vi "Square Pulse Fit Result String.vi"(8 "error in (no error)":errorcluster, 9 "Square Pulse Statistics":T3 {"Falling Edge Width" format="%0.2f"; "Rising Edge Width" format="%0.2f"; "Falling Edge Midpoint" format="%0.2f"; "Rising Edge Midpoint" format="%0.2f"; "Low Level" format="%0.2f"; "High Level" format="%0.2f"}, 10 "Square Pulse Options":T1={"Method"=enum."Mode", "# Bins"=0, "Threshold %"=10.0, "Center on Midpoint"=FALSE, "Smoothen Plot"=FALSE}, 11 "ROI Descriptor":T4 {"Contours"."Type" items=["No Selection", "Point", "Line", "Rectangle", "Oval", "Polygon", "Freehand Region", "Annulus", "Unused2", "Unused3", "Broken Line", "Freehand Line", "Rotated Rectangle"]}) -> (0 "error out":errorcluster, 3 "Result String":string)   [LabVIEW 2021, in "Fits.lvlib"]
uses:
  Fits.lvlib
  Square Pulse Statistics.ctl
  Square Pulse Options.ctl
  Square Pulse Levels Type.ctl
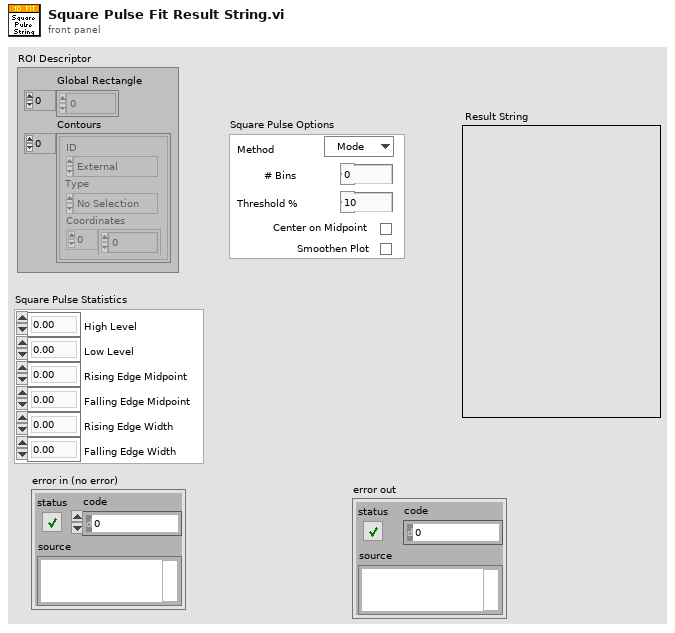
[diagram p1: front panel]
types:
  T1 = typedef "Fits.lvlib/Square Pulse Options.ctl" = cluster{"Method":T2, "# Bins":i32, "Threshold %":dbl, "Center on Midpoint":bool, "Smoothen Plot":bool}
  T2 = typedef "Fits.lvlib/Square Pulse Levels Type.ctl" = enum16{"Mode", "Mean"}
  T3 = typedef "Fits.lvlib/Square Pulse Statistics.ctl" = cluster{"High Level":dbl, "Low Level":dbl, "Rising Edge Midpoint":dbl, "Falling Edge Midpoint":dbl, "Rising Edge Width":dbl, "Falling Edge Width":dbl}
  T4 = typedef "ROI Descriptor" = cluster{"Global Rectangle":i32[], "Contours":cluster{"ID":enum32{"External", "Internal"}, "Type":u32, "Coordinates":i32[]}[]}
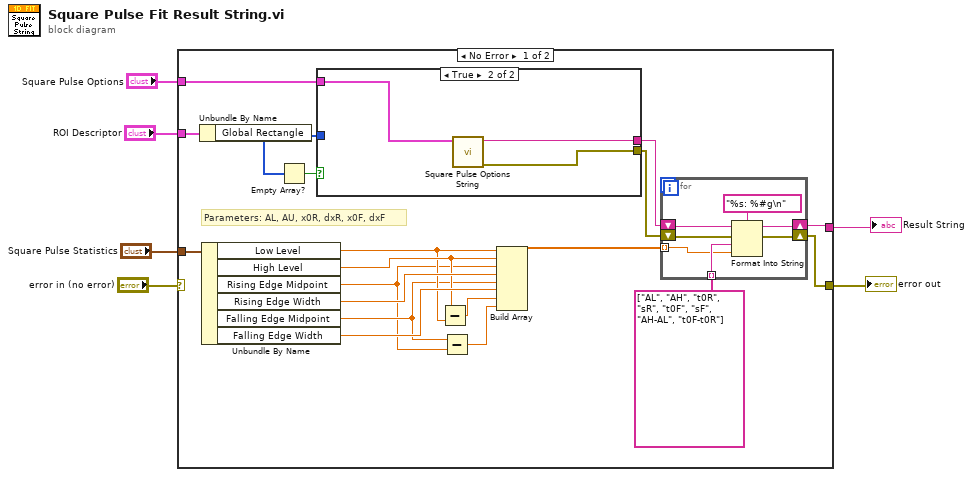
[diagram p0: block diagram]
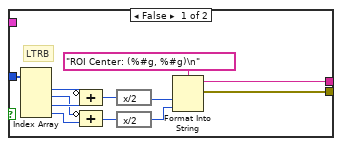
[diagram p2: hidden frame]
diagram:
  n1 = case shown="No Error" "error in (no error)" {
    selector: "error in (no error)" -> [_ w48]
    tunnel: [w21 w48] -> w5
    tunnel: "ROI Descriptor" -> [w25 _]
    tunnel: [w22 _] -> w3
    tunnel: "Square Pulse Statistics" -> [w17 _]
    tunnel: "Square Pulse Options" -> [w7 _]
    frame No Error {
      # "Parameters: AL, AU, x0R, dxR, x0F, dxF"
      n2 = Unbundle By Name(w25) -> ("Global Rectangle"=w20:i32[])
      n3 = Unbundle By Name(w17) -> ("Low Level"=w12:dbl, "High Level"=w13:dbl, "Rising Edge Midpoint"=w9:dbl, "Rising Edge Width"=w16:dbl, "Falling Edge Midpoint"=w10:dbl, "Falling Edge Width"=w15:dbl)
      n4 = Empty Array?(array=w20) -> (empty?=w19:bool)
      n5 = case shown="True" w19 {
        tunnel: [w28 w38] -> w24
        tunnel: [w27 w39] -> w23
        tunnel: w20 -> [w26 _]
        tunnel: w7 -> [_ w40]
        frame False {
          # "LTRB"
          n6 = Index Array(array=w26) -> (element #1=w37:i32, element #2=w34:i32, element #3=w36:i32, element #4=w35:i32)  [unwired: 4 in]
          n7 = Compound Arithmetic op=ADD(invert w37, w36) -> (w33:i32)
          n8 = Compound Arithmetic op=ADD(invert w34, w35) -> (w32:i32)
          n9 = expression code="x/2"(w33) -> (w30:i32)
          n10 = expression code="x/2"(w32) -> (w29:i32)
          n11 = Format Into String(format string="ROI Center: (%#g, %#g)\n", w30, w29) -> (resulting string=w27:string, error out=w28:errorcluster)  [unwired: 2 in]
        }
        frame True {
          n12 = call "Square Pulse Options String.vi"("Square Pulse Options"=w40) -> ("Error Out"=w38:errorcluster, "Option String"=w39:string)  [unwired: 9 in]
        }
      }
      n13 = Subtract(x=w13, y=w12) -> (x-y=w11:dbl)
      n14 = Subtract(x=w10, y=w9) -> (x-y=w8:dbl)
      n15 = Build Array(w12, w13, w9, w16, w10, w15, w11, w8) -> (w14:dbl[])
      n16 = for {
        tunnel: w14 -> [w41] mode=indexing
        shift-right: [w45] -> w22
        shift-left: w23 -> [w46]
        shift-right: [w44] -> w21
        shift-left: w24 -> [w43]
        tunnel: string[] ["AL", "AH", "t0R", "sR", "t0F", "sF", "AH-AL", "t0F-t0R"] -> [w42] mode=indexing
        n17 = Format Into String(format string="%s: %#g\n", initial string=w46, error in=w43, w42, w41) -> (resulting string=w45:string, error out=w44:errorcluster)
      }
    }
    frame Error {
    }
  }
  "Result String" <- w3
  "error out" <- w5
